vi "NACA_0015_Pressure.vi"(3 "Mode":T5, 5 "Traverse line In":T1 {"Row Duration (mins)" format="%#.1f"; "Row No" min=0; "Trace Gas Concentration (%)" min=0.0 format="%#.2f"; "Emission Rate (l/min)" format="%#.2f"; "Tunnel Speed" format="%#.2f"; "Start X" format="%#.2f"; "Start Y" format="%#.2f"; "Start Z" format="%#.2f"; "End X" format="%#.2f"; "End Y" format="%#.2f"; "End Z" format="%#.2f"; "Averaging time (min)" min=0.0 format="%#.2f"}) -> (0 "Error Message":string, 1 "Status":T4, 2 "Traverse line Out":T1 {"Row Duration (mins)" format="%#.1f"; "Row No" min=0; "Trace Gas Concentration (%)" min=0.0 format="%#.2f"; "Emission Rate (l/min)" format="%#.2f"; "Tunnel Speed" format="%#.2f"; "Start X" format="%#.2f"; "Start Y" format="%#.2f"; "Start Z" format="%#.2f"; "End X" format="%#.2f"; "End Y" format="%#.2f"; "End Z" format="%#.2f"; "Averaging time (min)" min=0.0 format="%#.2f"})   [LabVIEW 2011]
uses:
  Gen Trav/Traverse_cluster.ctl
  Gen Trav/Spacing.ctl
  Controls/Multi_run_mode.ctl
  Controls/User_Specific_mode.ctl
  Gen Trav/Multi_Run_Status.ctl
  Controls/Save_Data.ctl
  Controls/Setup.ctl
  <vilib>/Analysis/1siggen.llb/Ramp Pattern by Delta.vi
  Globals/Trav_pos_global.vi
  Globals/Extra_Commands_Global.vi
  Globals/Meas_global.vi
  <vilib>/Analysis/NI_AALBase.lvlib
panel:
  in  "stop":bool
  out "XY Graph":cluster{dbl[], dbl[]}(graph)
  out "Measurement No":i32
  # "X           Y            Z"
  # "Start"
  # "End"
  # "X           Y            Z"
  # "Start"
  # "End"
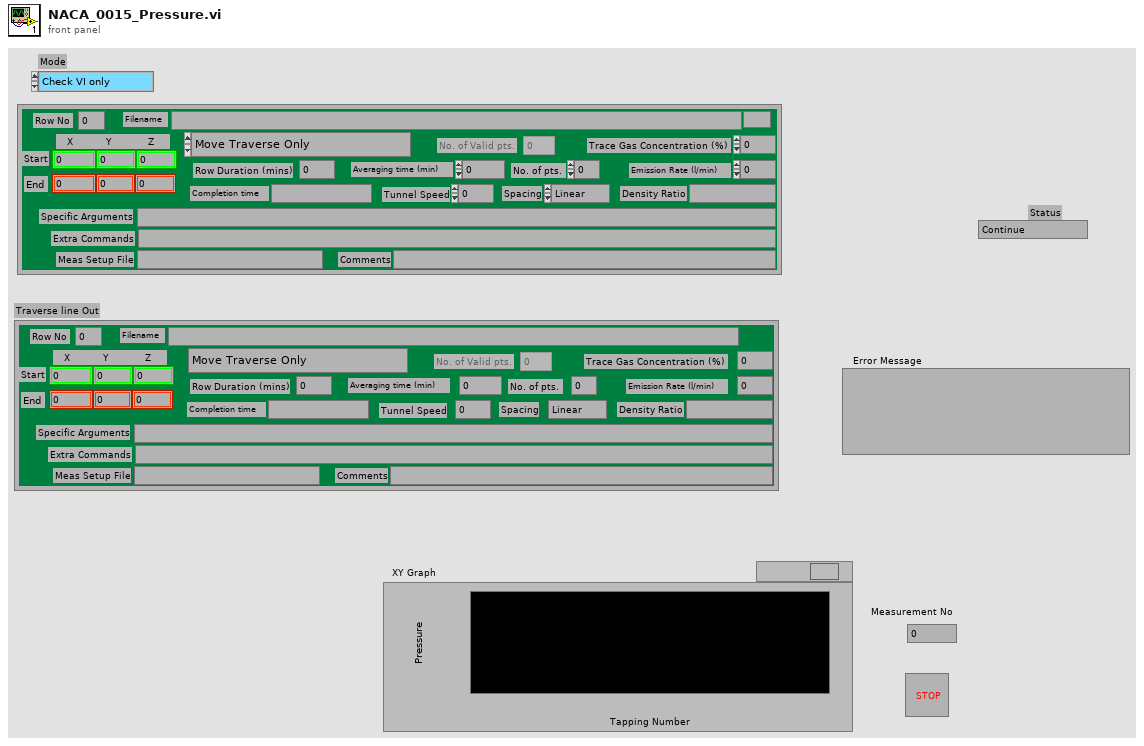
[diagram p1: front panel]
types:
  T1 = typedef "Traverse_cluster.ctl" = cluster{"Start X":dbl, "Start Y":dbl, "Start Z":dbl, "End X":dbl, "End Y":dbl, "End Z":dbl, "No. of pts.":i32, "Spacing":T2, "Filename":path, "Tunnel Speed":dbl, "Averaging time (min)":dbl, "Extra Commands":string, "Specific Arguments":string, "Emission Rate (l/min)":dbl, "Trace Gas Concentration (%)":dbl, "Density Ratio":string, "Comments":string, "Row No":i32, "Row Type Selector":T3, "Completion time":string, "Row Duration (mins)":dbl, "No. of Valid pts.":i32, "Meas Setup File":string}
  T2 = typedef "Spacing.ctl" = enum16{"Linear", "Log", "Gauss", "Specified", "N/A"}
  T3 = typedef "Multi_run_mode.ctl" = enum16{"Move Traverse Only", "Set Tunnel Speed Only", "Set Source Only", "Set Measurement Conditions", "Single Measurement", "Vertical Profile", "Lateral Profile", "Longitudinal Profile", "Explore Volume", "Multi-Axis Profile", "Auto Calibrate", "Meas Fast FID Bkgnd", "Check Beam Power", "Scanning Valve Measurement", "Run VI Named:", "Set ADAM Ch", "Wait (minutes)", "Send Message", "Synchronize With:", "Fall Back to this Row", "Turn Off Row Repeating", "Blank Row", "Traverse 3D Volume"}
  T4 = typedef "Multi_Run_Status.ctl" = enum16{"Continue", "Jump to Next Point", "Jump to Next Row", "Jump To Fall Back", "Terminate Run"}
  T5 = typedef "User_Specific_mode.ctl" = enum16{"Check VI only", "Run VI"}
  T6 = typedef "Save_Data.ctl" = enum16{"Save No Data", "Save Data"}
  T7 = typedef "Setup.ctl" = enum16{"Run Program", "Show Setup", "Save Current Setup", "Setup Front Panel"}
  T8 = cluster{"Name":string, "X":dbl, "Y":dbl, "Z":dbl}[]
  T9 = cluster{"Name":string, "X":dbl, "Y":dbl, "Z":dbl}
  T10 = typedef "Status_Cluster.ctl" = cluster{"Status":T4, "Error Type":string, "Error Description":string}
  T11 = typedef "Velocity_cluster.ctl" = cluster{"Name":string, "U":dbl, "u^2":dbl, "u^3/(u^2)^(1.5)":dbl, "u^4/(u^2)^2 -3":dbl, "% u'/U":dbl, "Mean % Err":dbl, "u^4":dbl}
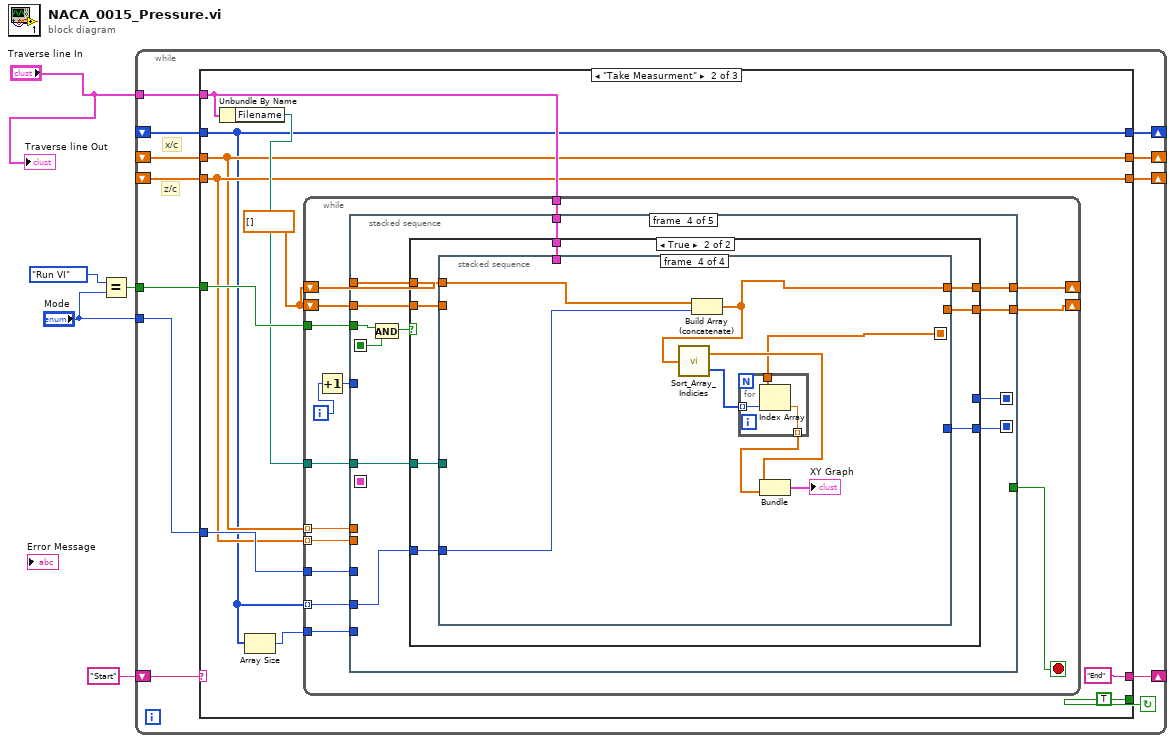
[diagram p0: block diagram]
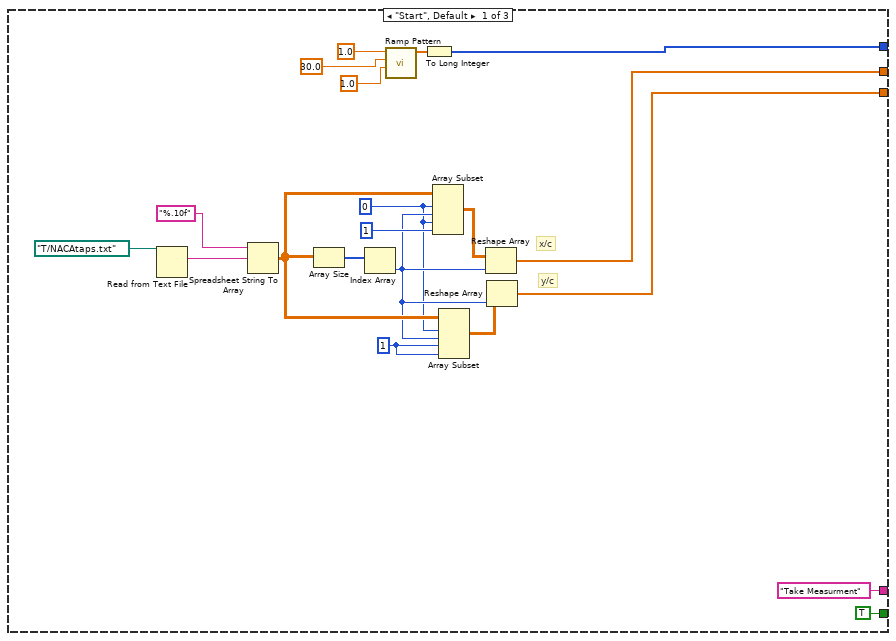
[diagram p2: hidden frame]
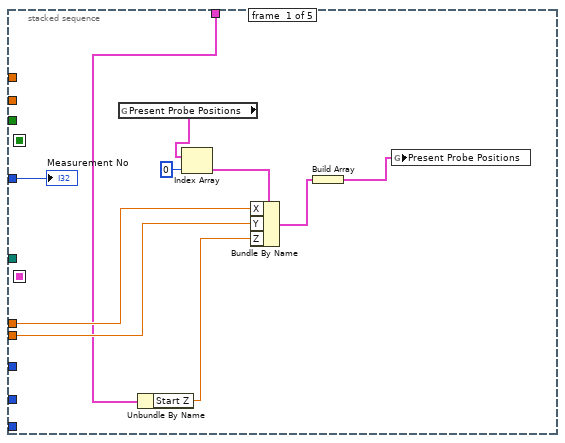
[diagram p3: hidden frame]
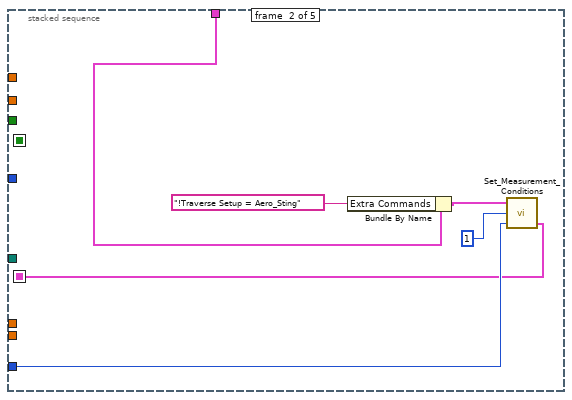
[diagram p4: hidden frame]
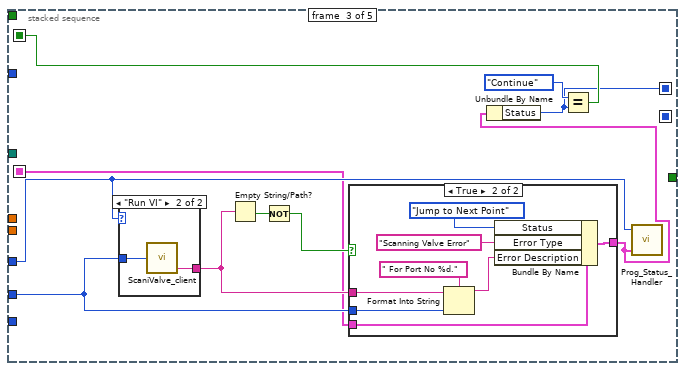
[diagram p5: hidden frame]
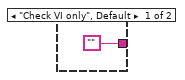
[diagram p6: hidden frame]
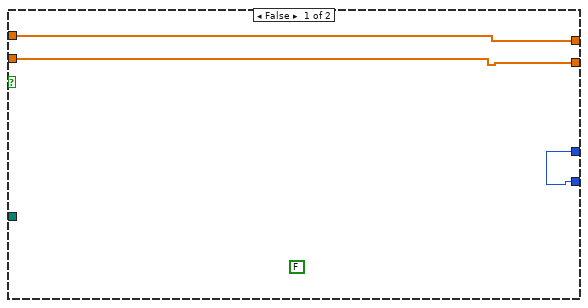
[diagram p8: hidden frame]
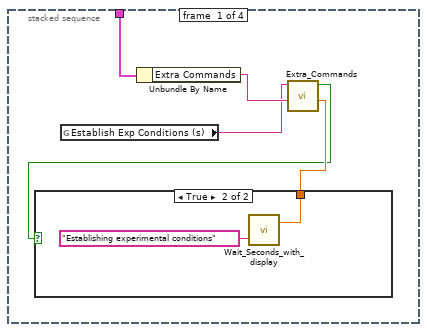
[diagram p9: hidden frame]
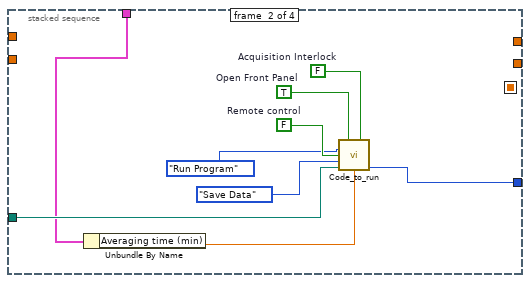
[diagram p11: hidden frame]
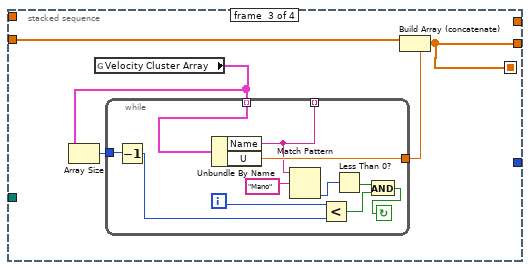
[diagram p12: hidden frame]
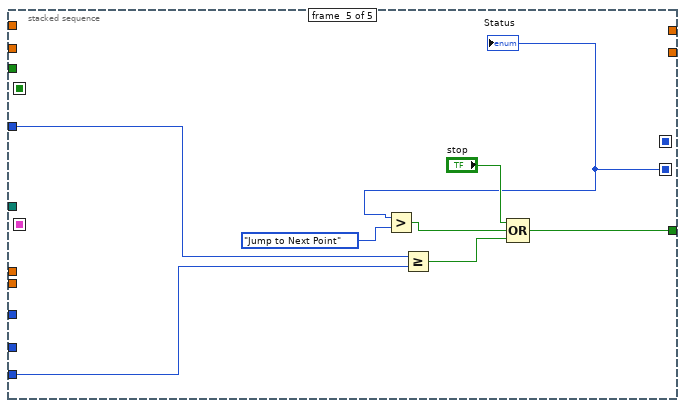
[diagram p13: hidden frame]
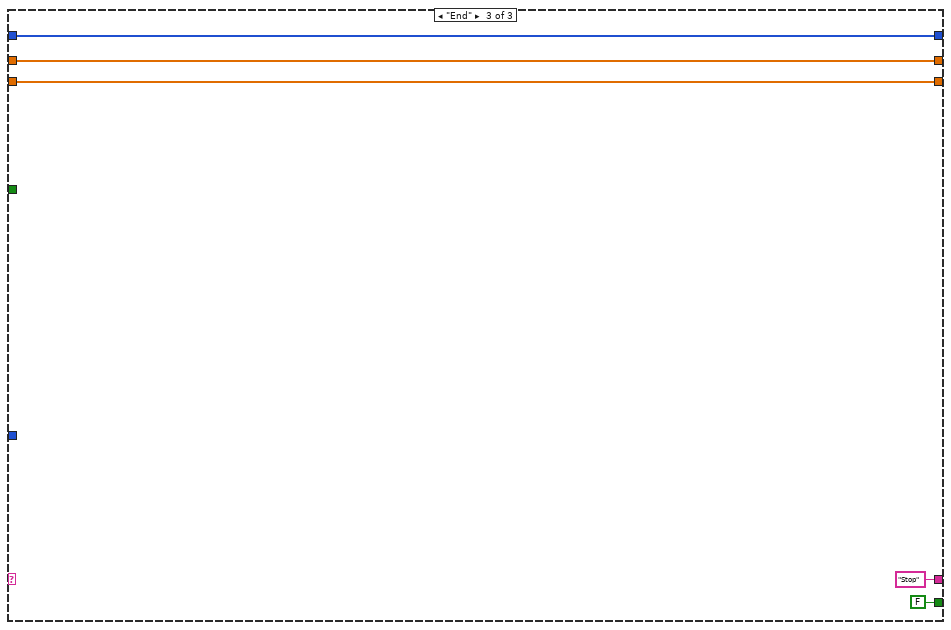
[diagram p14: hidden frame]
diagram:
  n1 = Equal?(x=User_Specific_mode."Run VI" ("Mode"), y="Mode") -> (x = y?=w2:bool)
  n2 = while {
    tunnel: "Traverse line In" -> [w16]
    shift-right: [w15] -> _
    shift-left: "Start" -> [w14]
    tunnel: "Mode" -> [w13]
    tunnel: w2 -> [w12]
    shift-right: [w11] -> _
    shift-left: _ -> [w10]
    shift-right: [w9] -> _
    shift-left: _ -> [w7]
    shift-right: [w8] -> _
    shift-left: _ -> [w6]
    stop <- w17 continue-if-true
    # "z/c"
    # "x/c"
    n3 = case shown="\"Take Measurment\"" w14 {
      tunnel: [TRUE TRUE FALSE] -> w17
      tunnel: w16 -> [_ w44 _]
      tunnel: ["Take Measurment" "End" "Stop"] -> w15
      tunnel: w13 -> [_ w42 _]
      tunnel: w12 -> [_ w45 _]
      tunnel: [w33 w39 w178] -> w11
      tunnel: w10 -> [_ w39 w178]
      tunnel: [w19 w40 w177] -> w9
      tunnel: [w18 w41 w176] -> w8
      tunnel: w7 -> [_ w40 w177]
      tunnel: w6 -> [_ w41 w176]
      frame "Start", Default {
        w20 = 1 ("index")
        w21 = 0 ("index")
        # "y/c"
        # "x/c"
        n4 = Read from Text File(file (use dialog)=path "T:/NACAtaps.txt") -> (text=w29:string)  [unwired: 3 in, 3 out]
        n5 = Spreadsheet String To Array(format string="%.10f", spreadsheet string=w29) -> (array=w25:dbl[][])  [unwired: 2 in]
        n6 = Array Size(array=w25) -> (size(s)=w27:i32[])
        n7 = Index Array(array=w27) -> (element=w22:i32)  [unwired: 1 in]
        n8 = call-poly <vilib>:"Ramp Pattern.vi"("start"=1.0, "end"=30.0, "delta"=1.0) -> ("Ramp Pattern"=w37:dbl[])  [unwired: 6 in, 2 out]
        n9 = To Long Integer(number=w37) -> (32bit integer=w33:i32[])
        n10 = Array Subset(array=w25, index (row)=w21, length (row)=w22, index (col)=w21, length (col)=1 ("length")) -> (w24:dbl[][])
        n11 = Array Subset(array=w25, index (row)=w21, length (row)=w22, index (col)=w20, length (col)=w20) -> (w23:dbl[][])
        n12 = Reshape Array(w24, w22) -> (w19:dbl[])
        n13 = Reshape Array(w23, w22) -> (w18:dbl[])
      }
      frame "Take Measurment" {
        w46 = dbl[] []
        n14 = Unbundle By Name(w44) -> ("Filename"=w43:path)
        n15 = Array Size(array=w39) -> (size(s)=w38:i32)
        n16 = while {
          tunnel: w42 -> [w58]
          tunnel: w45 -> [w55]
          tunnel: w43 -> [w63]
          shift-right: [w61] -> _
          shift-left: w46 -> [w62]
          shift-right: [w59] -> _
          shift-left: w46 -> [w60]
          tunnel: w44 -> [w57]
          tunnel: w39 -> [w52] mode=indexing
          tunnel: w40 -> [w51] mode=indexing
          tunnel: w41 -> [w50] mode=indexing
          tunnel: w38 -> [w49]
          i -> [w54]
          stop <- w56 stop-if-true
          n17 = Increment(x=w54) -> (x+1=w53:i32)
          n18 = stacked-sequence {
            seq-local: [_ _ w83 _ _] -> [_ _ _ w105 _]
            seq-local: [_ _ w82 _ _] -> [_ _ _ w106 _]
            seq-local: [_ _ _ w107 _] -> [_ _ _ _ w169]
            seq-local: [_ w74 _ _ _] -> [_ _ w80 _ _]
            tunnel: w63 -> [_ _ _ w113 _]
            tunnel: w62 -> [_ _ _ w112 _]
            tunnel: [_ _ _ w111 _] -> w61
            tunnel: w60 -> [_ _ _ w110 _]
            tunnel: [_ _ _ w109 _] -> w59
            tunnel: w58 -> [_ w75 w86 _ _]
            tunnel: w57 -> [w67 w76 _ w108 _]
            tunnel: w53 -> [w73 _ _ _ w172]
            tunnel: [_ _ _ _ w170] -> w56
            tunnel: w55 -> [_ _ _ w104 _]
            tunnel: w52 -> [_ _ w81 w102 _]
            tunnel: w51 -> [w72 _ _ _ _]
            tunnel: w50 -> [w71 _ _ _ _]
            tunnel: w49 -> [_ _ _ _ w168]
            frame #0 {
              n19 = global read "Trav_pos_global.vi" "Present Probe Positions"() -> (w69:T8)
              n20 = Unbundle By Name(w67) -> ("Start Z"=w66:dbl)
              n21 = Index Array(array=w69, index=0) -> (element=w68:T9)
              n22 = Bundle By Name(cluster=w68, "X"=w72, "Y"=w71, "Z"=w66) -> (w65:T9)
              n23 = Build Array(w65) -> (w64:T8)
              n24 = global write "Trav_pos_global.vi" "Present Probe Positions"(w64) -> ()
              "Measurement No" <- w73
            }
            frame #1 {
              n25 = Bundle By Name(cluster=w76, "Extra Commands"="!Traverse Setup = Aero_Sting") -> (w79:T1)
              n26 = call "Set_Measurement_Conditions.vi"("Simulate/Run"=w75, "Currently on Point"=1, "Traverse line"=w79) -> ("Status Cluster"=w74:T10)  [unwired: 2 in]
            }
            frame #2 {
              n27 = case shown="\"Run VI\"" w86 {
                tunnel: w81 -> [_ w92]
                tunnel: ["" w91] -> w87
                frame "Check VI only", Default {
                }
                frame "Run VI" {
                  n28 = call "ScaniValve_client.vi"("Port Number"=w92) -> ("Error String"=w91:string)  [unwired: 2 out]
                }
              }
              n29 = Empty String/Path?(string/path=w87) -> (empty?=w89:bool)
              n30 = Not(x=w89) -> (.not. x?=w88:bool)
              n31 = case shown="True" w88 {
                tunnel: w80 -> [w93 w101]
                tunnel: [w93 w98] -> w84
                tunnel: w87 -> [_ w95]
                tunnel: w81 -> [_ w94]
                frame False {
                }
                frame True {
                  n32 = Format Into String(format string=" For Port No %d." ("Format String"), initial string=w95, w94) -> (resulting string=w96:string)  [unwired: 1 in, 1 out]
                  n33 = Bundle By Name(cluster=w101, "Status"=Multi_Run_Status."Jump to Next Point", "Error Type"="Scanning Valve Error" ("t"), "Error Description"=w96) -> (w98:T10)
                }
              }
              n34 = Unbundle By Name(w84) -> ("Status"=w82:T4)
              n35 = Equal?(x=Multi_Run_Status."Continue" ("Status"), y=w82) -> (x = y?=w83:bool)
              n36 = call "Prog_Status_Handler.vi"("Status Cluster"=w84, "Simulate/Run"=w86) -> ()  [unwired: 2 out]
            }
            frame #3 {
              n37 = And(x=w104, y=w105) -> (x .and. y?=w103:bool)
              n38 = case shown="True" w103 {
                tunnel: [w114 w124] -> w107
                tunnel: w113 -> [_ w123]
                tunnel: w112 -> [w116 w122]
                tunnel: [w116 w121] -> w111
                tunnel: w110 -> [w115 w120]
                tunnel: [w115 w119] -> w109
                tunnel: w108 -> [_ w118]
                tunnel: w102 -> [_ w117]
                tunnel: w106 -> [w114 _]
                frame False {
                  (unwired) FALSE ("stop")
                }
                frame True {
                  n39 = stacked-sequence {
                    seq-local: [_ _ w143 _] -> [_ _ _ w159]
                    tunnel: [_ w134 _ _] -> w124
                    tunnel: w123 -> [_ w133 _ _]
                    tunnel: w122 -> [_ _ w144 _]
                    tunnel: [_ _ w143 _] -> w121
                    tunnel: w120 -> [_ _ _ w164]
                    tunnel: [_ _ _ w162] -> w119
                    tunnel: w118 -> [w129 w132 _ _]
                    tunnel: w117 -> [_ _ _ w157]
                    frame #0 {
                      n40 = global read "Extra_Commands_Global.vi" "Establish Exp Conditions (s)"() -> (w126:string)
                      n41 = Unbundle By Name(w129) -> ("Extra Commands"=w128:string)
                      n42 = call "Extra_Commands.vi"("String to Search"=w128, "Command"=w126) -> ("Numeric Value"=w127:dbl, "Command Found"=w125:bool)  [unwired: 2 in, 2 out]
                      n43 = case shown="True" w125 {
                        tunnel: w127 -> [_ w131]
                        frame False {
                        }
                        frame True {
                          n44 = call "Wait_Seconds_with_display.vi"("Message"="Establishing experimental conditions", "Seconds to wait"=w131) -> ()  [unwired: 1 in, 1 out]
                        }
                      }
                    }
                    frame #1 {
                      w137 = FALSE  # Acquisition Interlock
                      w138 = TRUE  # Open Front Panel
                      w140 = FALSE  # Remote control
                      n45 = Unbundle By Name(w132) -> ("Averaging time (min)"=w139:dbl)
                      n46 = call "Code_to_run.vi"("Open Front Panel"=w138, "Acquisition Interlock"=w137, "setup"=Setup."Run Program", "Remote control"=w140, "File"=Save_Data."Save Data", "Results Filename"=w133, "Averaging time (min)"=w139) -> ("Status"=w134:T4)  [unwired: 4 in, 4 out]
                    }
                    frame #2 {
                      n47 = global read "Meas_global.vi" "Velocity Cluster Array"() -> (w142:T11[])
                      n48 = Array Size(array=w142) -> (size(s)=w141:i32)
                      n49 = while {
                        tunnel: w142 -> [w156] mode=indexing
                        tunnel: [w154] -> _ mode=indexing
                        tunnel: [w155] -> w145
                        tunnel: w141 -> [w151]
                        i -> [w152]
                        stop <- w146 continue-if-true
                        n50 = Decrement(x=w151) -> (x-1=w150:i32)
                        n51 = Unbundle By Name(w156) -> ("Name"=w154:string, "U"=w155:dbl)
                        n52 = Match Pattern(string=w154, regular expression="Mano") -> (offset past match=w149:i32)  [unwired: 4 out]
                        n53 = Less?(x=w152, y=w150) -> (x < y?=w147:bool)
                        n54 = Less Than 0?(x=w149) -> (x < 0?=w148:bool)
                        n55 = And(x=w148, y=w147) -> (x .and. y?=w146:bool)
                      }
                      n56 = Build Array (concatenate)(w144, w145) -> (w143:dbl[])
                    }
                    frame #3 {
                      n57 = Build Array (concatenate)(w164, w157) -> (w162:dbl[])
                      n58 = call "Sort_Array_Indicies.vi"("unsorted array"=w162) -> ("sorted array"=w161:dbl[], "Sort Index"=w160:i32[])
                      n59 = for {
                        tunnel: w160 -> [w167] mode=indexing
                        tunnel: w159 -> [w166]
                        tunnel: [w165] -> w158 mode=indexing
                        n60 = Index Array(array=w166, index=w167) -> (element=w165:dbl)
                      }
                      n61 = Bundle("sorted array"=w161, w158) -> (→"XY Graph":cluster{"sorted array":dbl[], dbl[]})  [unwired: 1 out]
                    }
                  }
                }
              }
            }
            frame #4 {
              n62 = Greater?(x=w169, y=Multi_Run_Status."Jump to Next Point" ("Status")) -> (0:w174:bool)
              n63 = Greater Or Equal?(x=w172, y=w168) -> (x >= y?=w173:bool)
              n64 = Compound Arithmetic op=OR("stop", w174, w173) -> (w170:bool)
              "Status" <- w169
            }
          }
        }
      }
      frame "End" {
      }
    }
  }
  "Traverse line Out" <- "Traverse line In"
